vi "Sort Corelated Arrays by Amplitude.vi"(6 "peaks/valleys":enum32{"Peaks", "Valleys"}(ring), 10 "Amplitudes":dbl[](array[numeric]), 11 "Locations":dbl[](array[numeric])) -> (2 "Amplitudes SORTED DESC":dbl[](array[numeric]), 3 "Locations Sorted":dbl[](array[numeric]))   [LabVIEW 2015]
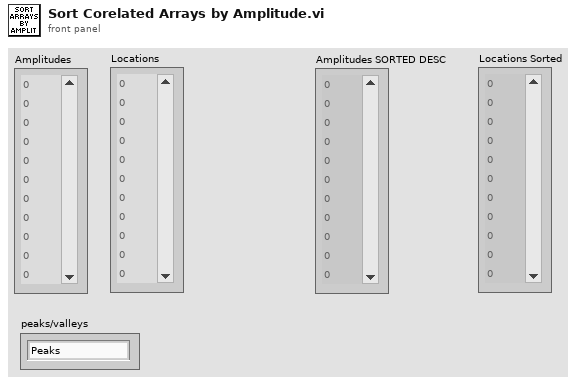
[diagram p1: front panel]
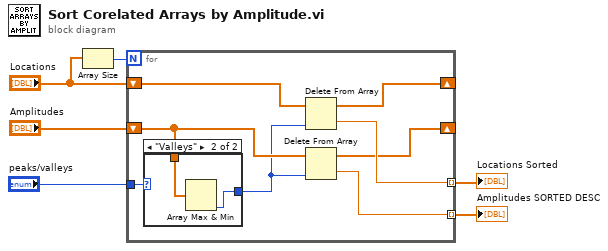
[diagram p0: block diagram]
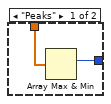
[diagram p2: hidden frame]
diagram:
  n1 = Array Size(array="Locations") -> (size(s)=w2:i32)
  n2 = for {
    N: w2 -> [_]
    shift-right: [w11] -> _
    shift-left: "Locations" -> [w14]
    shift-right: [w8] -> _
    shift-left: "Amplitudes" -> [w13]
    tunnel: [w10] -> w4 mode=indexing
    tunnel: [w9] -> w5 mode=indexing
    tunnel: "peaks/valleys" -> [w7]
    n3 = case shown="\"Valleys\"" w7 {
      tunnel: w13 -> [w16 w18]
      tunnel: [w15 w17] -> w12
      frame "Peaks" {
        n4 = Array Max & Min(array=w16) -> (max index (indices)=w15:i32)  [unwired: 3 out]
      }
      frame "Valleys" {
        n5 = Array Max & Min(array=w18) -> (min index (indices)=w17:i32)  [unwired: 3 out]
      }
    }
    n6 = Delete From Array(array=w14, index=w12) -> (deleted portion=w9:dbl, array with subset deleted=w11:dbl[])  [unwired: 1 in]
    n7 = Delete From Array(array=w13, index=w12) -> (deleted portion=w10:dbl, array with subset deleted=w8:dbl[])  [unwired: 1 in]
  }
  "Locations Sorted" <- w5
  "Amplitudes SORTED DESC" <- w4
